vi "Test_Good.vi"() -> ()   [LabVIEW 2018]
uses:
  <instrlib>/RIGOL DM3058/RIGOL DM3058.lvlib
panel:
  out "Measurement":dbl
  in  "VISA resource name":refnum<visa-resource-name>
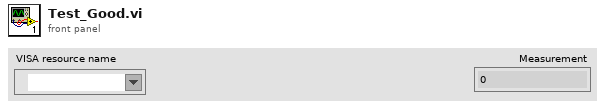
[diagram p1: front panel]
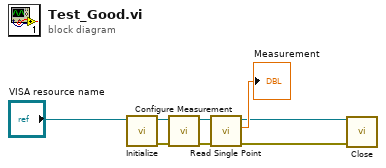
[diagram p0: block diagram]
diagram:
  n1 = call <instrlib>:"Initialize.vi"("VISA resource name"="VISA resource name") -> ("error out"=w4:errorcluster, "VISA resource name out"=w7:refnum<visa-resource-name>)  [unwired: 9 in]
  n2 = call <instrlib>:"Configure Measurement.vi"("error in (no error)"=w4, "VISA resource name"=w7) -> ("error out"=w3:errorcluster, "VISA resource name out"=w6:refnum<visa-resource-name>)  [unwired: 8 in]
  n3 = call <instrlib>:"Read Single Point.vi"("error in (no error)"=w3, "VISA resource name"=w6) -> ("error out"=w1:errorcluster, "Measurement"=→"Measurement":dbl, "VISA resource name out"=w2:refnum<visa-resource-name>)  [unwired: 7 in]
  n4 = call <instrlib>:"Close.vi"("error in (no error)"=w1, "VISA resource name"=w2) -> ()  [unwired: 9 in, 1 out]
